vi "Config Alarm.vi"(0 "VISA resource name":refnum<visa-resource-name>, 1 "Source (0: Kelvin)":u16(ring) items=["Kelvin", "Celsius", "Sensor Units", "Linear Data"], 2 "High Value (0.00)":dbl min=-100000.0 max=100000.0 step=0.01 format="%.2f", 5 "Input (0: A)":u16(ring) items=["A", "B", "C", "D"], 7 "Alarm On/Off (F: Alarm Off)":bool, 9 "Latch Enable (F: Disable Latch)":bool, 11 "error in (no error)":errorcluster, 12 "Relay Enable (F: Enable Relay)":bool, 13 "Low Value (0.00)":dbl min=-100000.0 max=100000.0 step=0.01 format="%.2f") -> (4 "VISA resource name out":refnum<visa-resource-name>, 15 "error out":errorcluster)   [LabVIEW 2020, in "Lake Shore Cryotronics 340.lvlib"]
doc: "This VI configures the alarm parameters for the 340's inputs."
uses:
  Lake Shore Cryotronics 340.lvlib
panel:
  # "Alarm On\nAlarm Off"
  # "Enable Latch\nDisable Latch"
  # "Enable Relay\nDisable Relay"
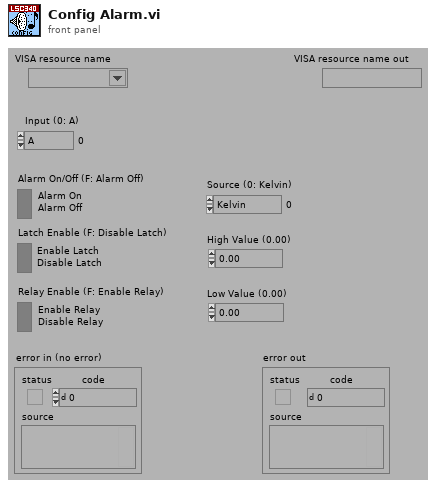
[diagram p1: front panel]
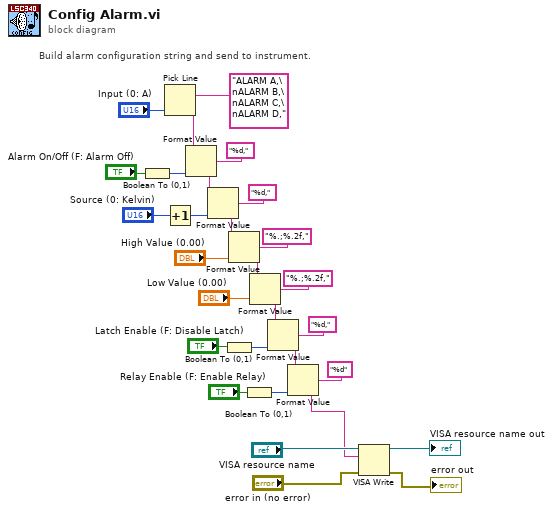
[diagram p0: block diagram]
diagram:
  # "Build alarm configuration string and send to instrument."
  n1 = Boolean To (0,1)(Boolean="Alarm On/Off (F: Alarm Off)") -> (0, 1=w25:i16)
  n2 = Pick Line(multi-line string="ALARM A,\nALARM B,\nALARM C,\nALARM D,", line index="Input (0: A)") -> (output string=w24:string)  [unwired: 1 in]
  n3 = Increment(x="Source (0: Kelvin)") -> (x+1=w21:u16)
  n4 = Format Value(string ("")=w24, format string="%d,", value (0)=w25) -> (output string=w20:string)
  n5 = Format Value(string ("")=w20, format string="%d,", value (0)=w21) -> (output string=w18:string)
  n6 = Boolean To (0,1)(Boolean="Latch Enable (F: Disable Latch)") -> (0, 1=w13:i16)
  n7 = Format Value(string ("")=w18, format string="%.;%.2f,", value (0)="High Value (0.00)") -> (output string=w15:string)
  n8 = Boolean To (0,1)(Boolean="Relay Enable (F: Enable Relay)") -> (0, 1=w10:i16)
  n9 = Format Value(string ("")=w15, format string="%.;%.2f,", value (0)="Low Value (0.00)") -> (output string=w7:string)
  n10 = Format Value(string ("")=w7, format string="%d,", value (0)=w13) -> (output string=w6:string)
  n11 = Format Value(string ("")=w6, format string="%d", value (0)=w10) -> (output string=w1:string)
  n12 = VISA Write(VISA resource name="VISA resource name", write buffer=w1, error in (no error)="error in (no error)") -> (VISA resource name out=→"VISA resource name out":refnum<visa-resource-name>, error out=→"error out":errorcluster)  [unwired: 1 out]
